vi "Get Caches.vi"(8 "error in (no error)":errorcluster, 11 "CPU Info in":refnum<class "CPU Hardware Info.lvclass">) -> (0 "error out":errorcluster, 2 "Caches":T1(array[cluster]), 3 "CPU Info out":refnum<class "CPU Hardware Info.lvclass">)   [LabVIEW 2017, in "Data Sharing Framework Core.lvlib" / "Data Sharing Framework Engine.lvlib" / "CPU Hardware Info.lvclass"]
uses:
  CPU Hardware Info.lvclass
  CPU Hardware Info.lvclass/CPU Hardware Info.ctl
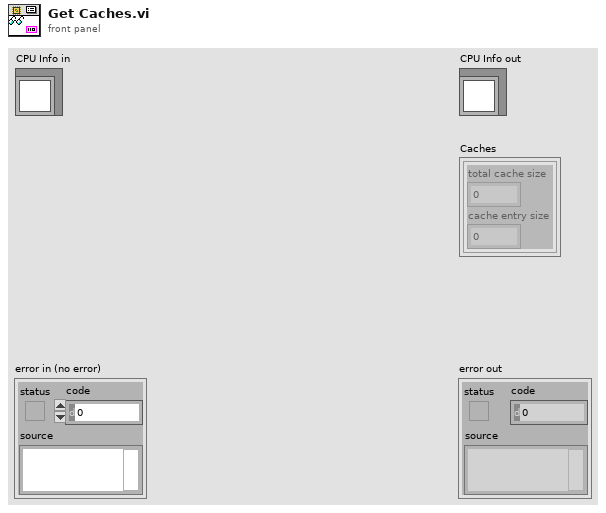
[diagram p1: front panel]
types:
  T1 = cluster{"total cache size":i32, "cache entry size":i32}[]
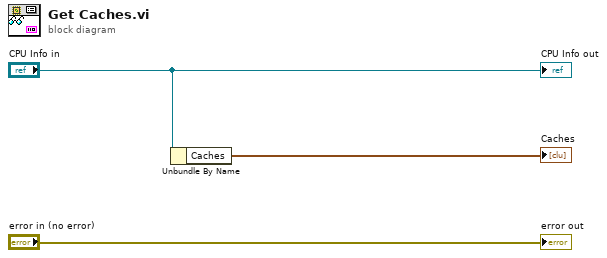
[diagram p0: block diagram]
diagram:
  n1 = Unbundle By Name("CPU Info in") -> ("Caches"=→"Caches":T1)
  "error out" <- "error in (no error)"
  "CPU Info out" <- "CPU Info in"
